vi "Subpanel_InitTree.vi"(0 "TreeControlRef":refnum<vi>, 5 "error in (no error)":errorcluster) -> (14 "TreeControlRef (out)":refnum<vi>, 19 "error out":errorcluster)   [LabVIEW 2016]
doc: "Initialisiert den Selection-Tree für die Subpanels.\n\n22.08.14 / sige"
uses:
  <vilib>/Utility/miscctls.llb/LVNodeAndColumnTypeDef.ctl
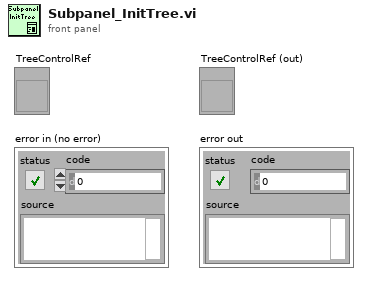
[diagram p1: front panel]
types:
  T1 = typedef "LVNodeAndColumnTypeDef.ctl" = cluster{"Node":string, "Column":i32}
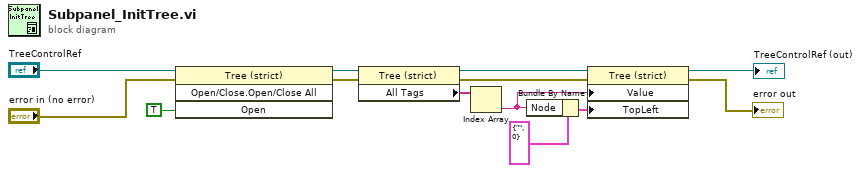
[diagram p0: block diagram]
diagram:
  n1 = invoke class="Tree (strict)" method="Open/Close.Open/Close All"(reference="TreeControlRef", error in="error in (no error)", "Open"=TRUE ("Open?")) -> (reference out=w4:refnum<vi>, error out=w2:errorcluster)  [unwired: 1 in, 2 out]
  n2 = property class="Tree (strict)"(reference=w4, error in=w2) -> (reference out=w6:refnum<vi>, error out=w1:errorcluster, "All Tags"=w7:string[])
  n3 = Index Array(array=w7) -> (element=w10:string)  [unwired: 1 in]
  n4 = Bundle By Name(cluster=T1 {"Node"="", "Column"=0} ("Top Left Visible Cell"), "Node"=w10) -> (w9:T1)
  n5 = property class="Tree (strict)"(reference=w6, error in=w1, "Value"=w10, "TopLeft"=w9) -> (reference out=→"TreeControlRef (out)":refnum<vi>, error out=→"error out":errorcluster)
